vi "Set Currents.vi"() -> (3 "DSM Message":string)   [LabVIEW 2016]
uses:
  Custom Pallet Controls/Custom Pallet Forward.ctl
  LabVIEW GEA2 Toolkit v1.0.0.0/library/GEA2_Toolkit.lvlib
panel:
  in  "UE Current (Amps x 10)":u16
  in  "LE Current (Amps x 10)":u16
  in  "Compressor Current (Amps x 10)":u16
  in  "No Load Current (Amps x 10)":u16
  out "Description":string="Set Currents"
  in  "Complete":T1
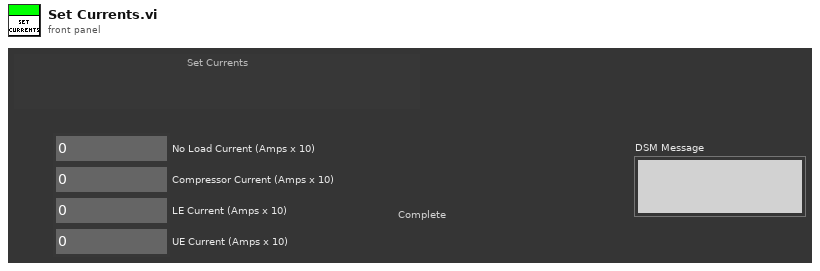
[diagram p1: front panel]
types:
  T1 = typedef "Custom Pallet Forward.ctl" = bool
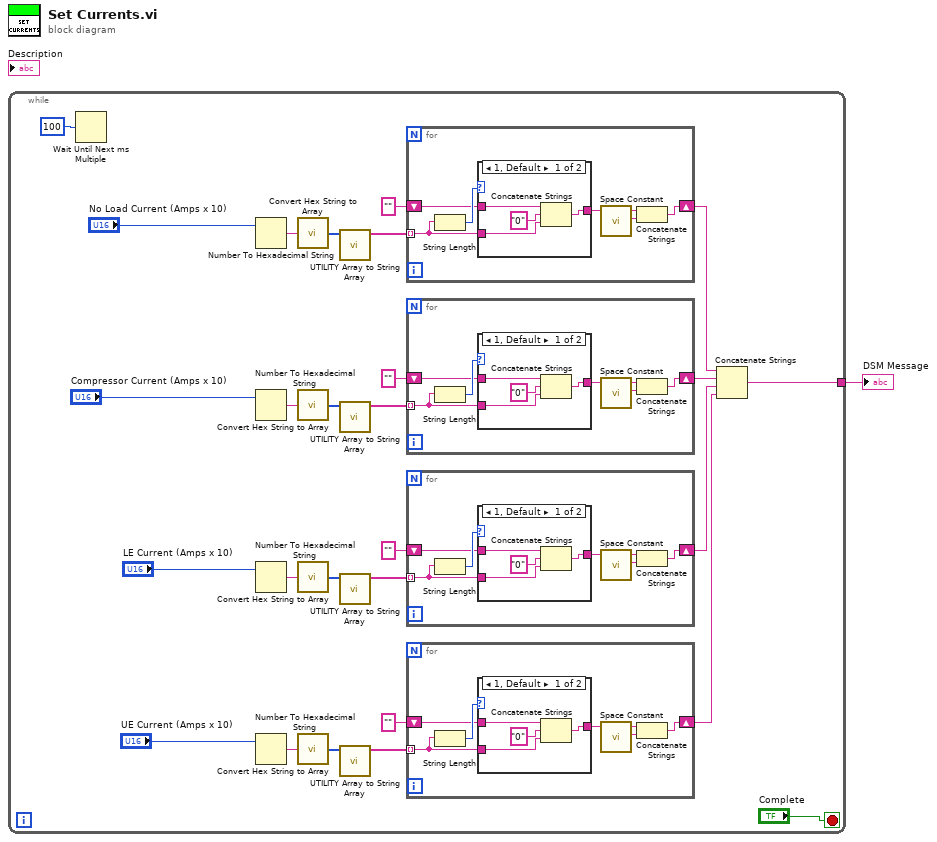
[diagram p0: block diagram]
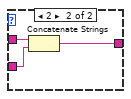
[diagram p2: hidden frame]
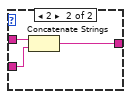
[diagram p3: hidden frame]
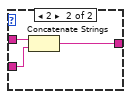
[diagram p4: hidden frame]
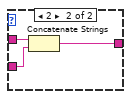
[diagram p5: hidden frame]
diagram:
  n1 = while {
    tunnel: [w13] -> w1
    stop <- "Complete" stop-if-true
    n2 = Wait Until Next ms Multiple(millisecond multiple=u32 100) -> ()  [unwired: 1 out]
    n3 = Number To Hexadecimal String(2:"No Load Current (Amps x 10)") -> (0:w25:string)  [unwired: 1 in]
    n4 = Number To Hexadecimal String(2:"Compressor Current (Amps x 10)") -> (0:w18:string)  [unwired: 1 in]
    n5 = Number To Hexadecimal String(2:"LE Current (Amps x 10)") -> (0:w20:string)  [unwired: 1 in]
    n6 = Number To Hexadecimal String(2:"UE Current (Amps x 10)") -> (0:w22:string)  [unwired: 1 in]
    n7 = call "Convert Hex String to Array.vi"("Hex String In"=w25) -> ("Hex Array Out"=w7:u8[])  [unwired: 14 in]
    n8 = call "Convert Hex String to Array.vi"("Hex String In"=w18) -> ("Hex Array Out"=w9:u8[])  [unwired: 14 in]
    n9 = call "Convert Hex String to Array.vi"("Hex String In"=w20) -> ("Hex Array Out"=w5:u8[])  [unwired: 14 in]
    n10 = call "Convert Hex String to Array.vi"("Hex String In"=w22) -> ("Hex Array Out"=w4:u8[])  [unwired: 14 in]
    n11 = call "UTILITY Array to String Array.vi"("Hex Array Out"=w7) -> ("Array"=w6:string[])  [unwired: 9 in, 1 out]
    n12 = call "UTILITY Array to String Array.vi"("Hex Array Out"=w9) -> ("Array"=w8:string[])  [unwired: 9 in, 1 out]
    n13 = call "UTILITY Array to String Array.vi"("Hex Array Out"=w5) -> ("Array"=w3:string[])  [unwired: 9 in, 1 out]
    n14 = call "UTILITY Array to String Array.vi"("Hex Array Out"=w4) -> ("Array"=w2:string[])  [unwired: 9 in, 1 out]
    n15 = for {
      tunnel: w6 -> [w71] mode=indexing
      shift-right: [w68] -> w17
      shift-left: "" -> [w72]
      n16 = String Length(string=w71) -> (length=w73:i32)
      n17 = case shown="1, Default" w73 {
        tunnel: w72 -> [w77 w80]
        tunnel: [w74 w79] -> w69
        tunnel: w71 -> [w75 w78]
        frame 1, Default {
          n18 = Concatenate Strings(w77, "0" ("string"), w75) -> (w74:string)
        }
        frame 2 {
          n19 = Concatenate Strings(w80, w78) -> (w79:string)
        }
      }
      n20 = call <vilib>:"Space Constant.vi"() -> ("String"=w70:string)
      n21 = Concatenate Strings(w69, w70) -> (w68:string)
    }
    n22 = for {
      tunnel: w8 -> [w58] mode=indexing
      shift-right: [w55] -> w16
      shift-left: "" -> [w59]
      n23 = String Length(string=w58) -> (length=w60:i32)
      n24 = case shown="1, Default" w60 {
        tunnel: w59 -> [w64 w67]
        tunnel: [w61 w66] -> w56
        tunnel: w58 -> [w62 w65]
        frame 1, Default {
          n25 = Concatenate Strings(w64, "0" ("string"), w62) -> (w61:string)
        }
        frame 2 {
          n26 = Concatenate Strings(w67, w65) -> (w66:string)
        }
      }
      n27 = call <vilib>:"Space Constant.vi"() -> ("String"=w57:string)
      n28 = Concatenate Strings(w56, w57) -> (w55:string)
    }
    n29 = for {
      tunnel: w3 -> [w45] mode=indexing
      shift-right: [w42] -> w15
      shift-left: "" -> [w46]
      n30 = String Length(string=w45) -> (length=w47:i32)
      n31 = case shown="1, Default" w47 {
        tunnel: w46 -> [w51 w54]
        tunnel: [w48 w53] -> w43
        tunnel: w45 -> [w49 w52]
        frame 1, Default {
          n32 = Concatenate Strings(w51, "0" ("string"), w49) -> (w48:string)
        }
        frame 2 {
          n33 = Concatenate Strings(w54, w52) -> (w53:string)
        }
      }
      n34 = call <vilib>:"Space Constant.vi"() -> ("String"=w44:string)
      n35 = Concatenate Strings(w43, w44) -> (w42:string)
    }
    n36 = for {
      tunnel: w2 -> [w32] mode=indexing
      shift-right: [w29] -> w14
      shift-left: "" -> [w33]
      n37 = String Length(string=w32) -> (length=w34:i32)
      n38 = case shown="1, Default" w34 {
        tunnel: w33 -> [w38 w41]
        tunnel: [w35 w40] -> w30
        tunnel: w32 -> [w36 w39]
        frame 1, Default {
          n39 = Concatenate Strings(w38, "0" ("string"), w36) -> (w35:string)
        }
        frame 2 {
          n40 = Concatenate Strings(w41, w39) -> (w40:string)
        }
      }
      n41 = call <vilib>:"Space Constant.vi"() -> ("String"=w31:string)
      n42 = Concatenate Strings(w30, w31) -> (w29:string)
    }
    n43 = Concatenate Strings(w17, w16, w15, w14) -> (w13:string)
  }
  "DSM Message" <- w1
